vi "诊断标定3 - 副本.vi"(8 "CAN端口":u16(ring), 9 "设备索引号":u16(ring), 10 "CAN卡类型":u32(ring)=21) -> ()   [LabVIEW 2013] (continued)
                n961 = property on="项目信息" class="Tbl (严格)"("Disabled"=w1279) -> ()  [unwired: 2 in, 2 out]
                n962 = global read "功能码全局.vi" "主板项目信息5"() -> (w1287:bool[])
                n963 = global read "功能码全局.vi" "主板项目信息6"() -> (w1285:bool[])
                n964 = Index Array(array=w1287, index=4 ("索引")) -> (element=w1283:bool)
                n965 = Index Array(array=w1285, index=5 ("索引")) -> (element=w1284:bool)
                n966 = Not(x=w1293) -> (.not. x?=w1292:bool)
              }
              frame "温度起始值" {
                w1329 = 2
                w1331 = FALSE
                n967 = property on="电池实际容量(A)" class="DigNum (严格)"("Disabled"=w1329) -> ()  [unwired: 2 in, 2 out]
                n968 = property on="使用者" class="DigNum (严格)"("Disabled"=w1329) -> ()  [unwired: 2 in, 2 out]
                n969 = property on="SOH(%)" class="DigNum (严格)"("Disabled"=w1329) -> ()  [unwired: 2 in, 2 out]
                n970 = property on="电池额定容量(A)" class="DigNum (严格)"("Disabled"=w1329) -> ()  [unwired: 2 in, 2 out]
                n971 = property on="SOC(%)" class="DigNum (严格)"("Disabled"=w1329) -> ()  [unwired: 2 in, 2 out]
                n972 = local read "从板个数"() -> (w1327:dbl)
                n973 = property on="系统时钟" class="Str"("Disabled"=w1329) -> ()  [unwired: 2 in, 2 out]
                n974 = property on="配置文件版本" class="Str"("Disabled"=w1329) -> ()  [unwired: 2 in, 2 out]
                n975 = property on="车架(牌)号" class="Str"("Disabled"=w1329) -> ()  [unwired: 2 in, 2 out]
                n976 = property on="产品编号" class="Str"("Disabled"=w1329) -> ()  [unwired: 2 in, 2 out]
                n977 = control-ref of="项目信息"() -> (w1328:refnum<vi>)
                n978 = stacked-sequence {
                  tunnel: w1328 -> [w1340 w1343 w1356]
                  tunnel: w1327 -> [w1333 w1342 w1355]
                  frame #0 {
                    n979 = Multiply(x=w1333, y=3.0) -> (x*y=w1335:dbl)
                    n980 = Compound Arithmetic op=ADD(23.0 ("值"), w1335) -> (w1337:dbl)
                    n981 = Bundle(w1337, 0) -> (w1339:cluster{dbl, i32})  [unwired: 1 out]
                    n982 = property class="Tbl (严格)"(reference=w1340, "Index Values"=w1339) -> ()  [unwired: 1 in, 2 out]
                  }
                  frame #1 {
                    n983 = for {
                      N: 10 -> [_]
                      tunnel: w1343 -> [w1353]
                      tunnel: w1342 -> [w1348]
                      i -> [w1347]
                      n984 = Multiply(x=4.0, y=w1348) -> (x*y=w1345:dbl)
                      n985 = Compound Arithmetic op=ADD(24.0 ("值"), w1345, w1347) -> (w1350:dbl)
                      n986 = Bundle(w1350, 0) -> (w1352:cluster{dbl, i32})  [unwired: 1 out]
                      n987 = property class="Tbl (严格)"(reference=w1353, "Active Cell"=w1352, "Cell BG Color"=u32 16448250) -> ()  [unwired: 1 in, 2 out]
                    }
                  }
                  frame #2 {
                    n988 = Increment(x=w1355) -> (x+1=w1354:dbl)
                    n989 = for {
                      N: w1354 -> [_]
                      tunnel: w1356 -> [w1366]
                      tunnel: w1355 -> [w1361]
                      i -> [w1360]
                      n990 = Multiply(x=3.0, y=w1361) -> (x*y=w1358:dbl)
                      n991 = Compound Arithmetic op=ADD(23.0 ("值"), w1358, w1360) -> (w1363:dbl)
                      n992 = Bundle(w1363, 0) -> (w1365:cluster{dbl, i32})  [unwired: 1 out]
                      n993 = property class="Tbl (严格)"(reference=w1366, "Active Cell"=w1365, "Cell BG Color"=u32 6618880) -> ()  [unwired: 1 in, 2 out]
                    }
                  }
                }
                n994 = Select(t=0, s=w1318, f=1) -> (s? t:f=w1317:i32)
                n995 = property on="从板个数" class="DigNum (严格)"("NumText.BGColor"=u32 13816530) -> ()  [unwired: 2 in, 2 out]
                n996 = property on="项目信息" class="Tbl (严格)"("Disabled"=w1317) -> ()  [unwired: 2 in, 2 out]
                n997 = global read "功能码全局.vi" "主板项目信息5"() -> (w1325:bool[])
                n998 = global read "功能码全局.vi" "主板项目信息6"() -> (w1323:bool[])
                n999 = Index Array(array=w1325, index=5 ("索引")) -> (element=w1322:bool)
                n1000 = Index Array(array=w1323, index=6 ("索引")) -> (element=w1321:bool)
                n1001 = Not(x=w1331) -> (.not. x?=w1330:bool)
              }
              frame "保险位置" {
                w1379 = 2
                w1381 = FALSE
                n1002 = property on="电池实际容量(A)" class="DigNum (严格)"("Disabled"=w1379) -> ()  [unwired: 2 in, 2 out]
                n1003 = property on="使用者" class="DigNum (严格)"("Disabled"=w1379) -> ()  [unwired: 2 in, 2 out]
                n1004 = property on="SOH(%)" class="DigNum (严格)"("Disabled"=w1379) -> ()  [unwired: 2 in, 2 out]
                n1005 = property on="电池额定容量(A)" class="DigNum (严格)"("Disabled"=w1379) -> ()  [unwired: 2 in, 2 out]
                n1006 = property on="SOC(%)" class="DigNum (严格)"("Disabled"=w1379) -> ()  [unwired: 2 in, 2 out]
                n1007 = local read "从板个数"() -> (w1377:dbl)
                n1008 = property on="系统时钟" class="Str"("Disabled"=w1379) -> ()  [unwired: 2 in, 2 out]
                n1009 = property on="配置文件版本" class="Str"("Disabled"=w1379) -> ()  [unwired: 2 in, 2 out]
                n1010 = property on="车架(牌)号" class="Str"("Disabled"=w1379) -> ()  [unwired: 2 in, 2 out]
                n1011 = property on="产品编号" class="Str"("Disabled"=w1379) -> ()  [unwired: 2 in, 2 out]
                n1012 = control-ref of="项目信息"() -> (w1378:refnum<vi>)
                n1013 = stacked-sequence {
                  tunnel: w1378 -> [w1390 w1393]
                  tunnel: w1377 -> [w1383 w1392]
                  frame #0 {
                    n1014 = Multiply(x=w1383, y=4.0) -> (x*y=w1385:dbl)
                    n1015 = Compound Arithmetic op=ADD(24.0 ("值"), w1385) -> (w1387:dbl)
                    n1016 = Bundle(w1387, 0) -> (w1389:cluster{dbl, i32})  [unwired: 1 out]
                    n1017 = property class="Tbl (严格)"(reference=w1390, "Index Values"=w1389) -> ()  [unwired: 1 in, 2 out]
                  }
                  frame #1 {
                    n1018 = for {
                      N: 20 -> [_]
                      tunnel: w1393 -> [w1403]
                      tunnel: w1392 -> [w1398]
                      i -> [w1397]
                      n1019 = Multiply(x=4.0, y=w1398) -> (x*y=w1395:dbl)
                      n1020 = Compound Arithmetic op=ADD(24.0 ("值"), w1395, w1397) -> (w1400:dbl)
                      n1021 = Bundle(w1400, 0) -> (w1402:cluster{dbl, i32})  [unwired: 1 out]
                      n1022 = property class="Tbl (严格)"(reference=w1403, "Active Cell"=w1402, "Cell BG Color"=u32 6618880) -> ()  [unwired: 1 in, 2 out]
                    }
                  }
                }
                n1023 = property on="从板个数" class="DigNum (严格)"("NumText.BGColor"=u32 13816530) -> ()  [unwired: 2 in, 2 out]
                n1024 = Select(t=0, s=w1370, f=1) -> (s? t:f=w1368:i32)
                n1025 = global read "功能码全局.vi" "主板项目信息4"() -> (w1375:bool[])
                n1026 = property on="项目信息" class="Tbl (严格)"("Disabled"=w1368) -> ()  [unwired: 2 in, 2 out]
                n1027 = Index Array(array=w1375, index #1=5 ("索引"), index #2=6 ("索引")) -> (element #1=w1373:bool, element #2=w1372:bool)
                n1028 = Not(x=w1381) -> (.not. x?=w1380:bool)
              }
              frame "SOC" {
                w1414 = 2
                w1416 = FALSE
                n1029 = property on="电池实际容量(A)" class="DigNum (严格)"("Disabled"=w1414) -> ()  [unwired: 2 in, 2 out]
                n1030 = property on="使用者" class="DigNum (严格)"("Disabled"=w1414) -> ()  [unwired: 2 in, 2 out]
                n1031 = property on="SOH(%)" class="DigNum (严格)"("Disabled"=w1414) -> ()  [unwired: 2 in, 2 out]
                n1032 = property on="电池额定容量(A)" class="DigNum (严格)"("Disabled"=w1414) -> ()  [unwired: 2 in, 2 out]
                n1033 = property on="从板个数" class="DigNum (严格)"("NumText.BGColor"=u32 13816530) -> ()  [unwired: 2 in, 2 out]
                n1034 = property on="系统时钟" class="Str"("Disabled"=w1414) -> ()  [unwired: 2 in, 2 out]
                n1035 = property on="配置文件版本" class="Str"("Disabled"=w1414) -> ()  [unwired: 2 in, 2 out]
                n1036 = property on="车架(牌)号" class="Str"("Disabled"=w1414) -> ()  [unwired: 2 in, 2 out]
                n1037 = property on="项目信息" class="Tbl (严格)"("Disabled"=w1414) -> ()  [unwired: 2 in, 2 out]
                n1038 = property on="产品编号" class="Str"("Disabled"=w1414) -> ()  [unwired: 2 in, 2 out]
                n1039 = Select(t=0, s=w1406, f=0) -> (s? t:f=w1405:i32)
                n1040 = property on="SOC(%)" class="DigNum (严格)"("Disabled"=w1405) -> ()  [unwired: 2 in, 2 out]
                n1041 = property on="项目信息2" class="Clust (严格)"("DisabledEnum"=w1405) -> ()  [unwired: 2 in, 2 out]
                n1042 = global read "功能码全局.vi" "主板项目信息7"() -> (w1412:bool[])
                n1043 = Index Array(array=w1412, index #1=2 ("索引"), index #2=5 ("索引")) -> (element #1=w1410:bool, element #2=w1409:bool)
                n1044 = Not(x=w1416) -> (.not. x?=w1415:bool)
              }
              frame "电池额定实际容量" {
                w1428 = 2
                w1430 = FALSE
                n1045 = property on="使用者" class="DigNum (严格)"("Disabled"=w1428) -> ()  [unwired: 2 in, 2 out]
                n1046 = property on="SOH(%)" class="DigNum (严格)"("Disabled"=w1428) -> ()  [unwired: 2 in, 2 out]
                n1047 = property on="SOC(%)" class="DigNum (严格)"("Disabled"=w1428) -> ()  [unwired: 2 in, 2 out]
                n1048 = property on="从板个数" class="DigNum (严格)"("NumText.BGColor"=u32 13816530) -> ()  [unwired: 2 in, 2 out]
                n1049 = property on="系统时钟" class="Str"("Disabled"=w1428) -> ()  [unwired: 2 in, 2 out]
                n1050 = property on="配置文件版本" class="Str"("Disabled"=w1428) -> ()  [unwired: 2 in, 2 out]
                n1051 = property on="车架(牌)号" class="Str"("Disabled"=w1428) -> ()  [unwired: 2 in, 2 out]
                n1052 = property on="项目信息" class="Tbl (严格)"("Disabled"=w1428) -> ()  [unwired: 2 in, 2 out]
                n1053 = property on="产品编号" class="Str"("Disabled"=w1428) -> ()  [unwired: 2 in, 2 out]
                n1054 = Select(t=0, s=w1420, f=1) -> (s? t:f=w1419:i32)
                n1055 = property on="电池实际容量(A)" class="DigNum (严格)"("Disabled"=w1419) -> ()  [unwired: 2 in, 2 out]
                n1056 = property on="电池额定容量(A)" class="DigNum (严格)"("Disabled"=w1419) -> ()  [unwired: 2 in, 2 out]
                n1057 = property on="项目信息2" class="Clust (严格)"("DisabledEnum"=w1419) -> ()  [unwired: 2 in, 2 out]
                n1058 = global read "功能码全局.vi" "主板项目信息7"() -> (w1426:bool[])
                n1059 = Index Array(array=w1426, index #1=3 ("索引"), index #2=6 ("索引")) -> (element #1=w1424:bool, element #2=w1423:bool)
                n1060 = Not(x=w1430) -> (.not. x?=w1429:bool)
              }
              frame "配置文件版本" {
                w1443 = 2
                w1445 = FALSE
                n1061 = property on="使用者" class="DigNum (严格)"("Disabled"=w1443) -> ()  [unwired: 2 in, 2 out]
                n1062 = property on="SOH(%)" class="DigNum (严格)"("Disabled"=w1443) -> ()  [unwired: 2 in, 2 out]
                n1063 = property on="SOC(%)" class="DigNum (严格)"("Disabled"=w1443) -> ()  [unwired: 2 in, 2 out]
                n1064 = property on="电池实际容量(A)" class="DigNum (严格)"("Disabled"=w1443) -> ()  [unwired: 2 in, 2 out]
                n1065 = property on="从板个数" class="DigNum (严格)"("NumText.BGColor"=u32 13816530) -> ()  [unwired: 2 in, 2 out]
                n1066 = property on="电池额定容量(A)" class="DigNum (严格)"("Disabled"=w1443) -> ()  [unwired: 2 in, 2 out]
                n1067 = property on="系统时钟" class="Str"("Disabled"=w1443) -> ()  [unwired: 2 in, 2 out]
                n1068 = property on="车架(牌)号" class="Str"("Disabled"=w1443) -> ()  [unwired: 2 in, 2 out]
                n1069 = property on="项目信息" class="Tbl (严格)"("Disabled"=w1443) -> ()  [unwired: 2 in, 2 out]
                n1070 = property on="产品编号" class="Str"("Disabled"=w1443) -> ()  [unwired: 2 in, 2 out]
                n1071 = Select(t=0, s=w1434, f=1) -> (s? t:f=w1433:i32)
                n1072 = property on="项目信息2" class="Clust (严格)"("DisabledEnum"=w1433) -> ()  [unwired: 2 in, 2 out]
                n1073 = property on="配置文件版本" class="Str"("Disabled"=w1433) -> ()  [unwired: 2 in, 2 out]
                n1074 = global read "功能码全局.vi" "主板项目信息5"() -> (w1441:bool[])
                n1075 = global read "功能码全局.vi" "主板项目信息6"() -> (w1440:bool[])
                n1076 = Index Array(array=w1441, index=6 ("索引")) -> (element=w1438:bool)
                n1077 = Index Array(array=w1440, index=7 ("索引")) -> (element=w1437:bool)
                n1078 = Not(x=w1445) -> (.not. x?=w1444:bool)
              }
              frame "参数修改记录" {
                w1458 = 2
                w1460 = FALSE
                n1079 = property on="SOH(%)" class="DigNum (严格)"("Disabled"=w1458) -> ()  [unwired: 2 in, 2 out]
                n1080 = property on="SOC(%)" class="DigNum (严格)"("Disabled"=w1458) -> ()  [unwired: 2 in, 2 out]
                n1081 = property on="电池实际容量(A)" class="DigNum (严格)"("Disabled"=w1458) -> ()  [unwired: 2 in, 2 out]
                n1082 = property on="电池额定容量(A)" class="DigNum (严格)"("Disabled"=w1458) -> ()  [unwired: 2 in, 2 out]
                n1083 = property on="从板个数" class="DigNum (严格)"("NumText.BGColor"=u32 13816530) -> ()  [unwired: 2 in, 2 out]
                n1084 = property on="系统时钟" class="Str"("Disabled"=w1458) -> ()  [unwired: 2 in, 2 out]
                n1085 = property on="车架(牌)号" class="Str"("Disabled"=w1458) -> ()  [unwired: 2 in, 2 out]
                n1086 = property on="配置文件版本" class="Str"("Disabled"=w1458) -> ()  [unwired: 2 in, 2 out]
                n1087 = property on="项目信息" class="Tbl (严格)"("Disabled"=w1458) -> ()  [unwired: 2 in, 2 out]
                n1088 = property on="产品编号" class="Str"("Disabled"=w1458) -> ()  [unwired: 2 in, 2 out]
                n1089 = Select(t=0, s=w1449, f=1) -> (s? t:f=w1448:i32)
                n1090 = property on="使用者" class="DigNum (严格)"("Disabled"=w1448) -> ()  [unwired: 2 in, 2 out]
                n1091 = property on="项目信息2" class="Clust (严格)"("DisabledEnum"=w1448) -> ()  [unwired: 2 in, 2 out]
                n1092 = global read "功能码全局.vi" "主板项目信息7"() -> (w1455:bool[])
                n1093 = global read "功能码全局.vi" "主板项目信息5"() -> (w1456:bool[])
                n1094 = Index Array(array=w1455, index=0 ("索引")) -> (element=w1453:bool)
                n1095 = Index Array(array=w1456, index=7 ("索引")) -> (element=w1452:bool)
                n1096 = Not(x=w1460) -> (.not. x?=w1459:bool)
              }
              frame "车牌号" {
                w1473 = 2
                w1475 = FALSE
                n1097 = property on="SOH(%)" class="DigNum (严格)"("Disabled"=w1473) -> ()  [unwired: 2 in, 2 out]
                n1098 = property on="使用者" class="DigNum (严格)"("Disabled"=w1473) -> ()  [unwired: 2 in, 2 out]
                n1099 = property on="SOC(%)" class="DigNum (严格)"("Disabled"=w1473) -> ()  [unwired: 2 in, 2 out]
                n1100 = property on="电池实际容量(A)" class="DigNum (严格)"("Disabled"=w1473) -> ()  [unwired: 2 in, 2 out]
                n1101 = property on="电池额定容量(A)" class="DigNum (严格)"("Disabled"=w1473) -> ()  [unwired: 2 in, 2 out]
                n1102 = property on="从板个数" class="DigNum (严格)"("NumText.BGColor"=u32 13816530) -> ()  [unwired: 2 in, 2 out]
                n1103 = property on="系统时钟" class="Str"("Disabled"=w1473) -> ()  [unwired: 2 in, 2 out]
                n1104 = property on="配置文件版本" class="Str"("Disabled"=w1473) -> ()  [unwired: 2 in, 2 out]
                n1105 = property on="项目信息" class="Tbl (严格)"("Disabled"=w1473) -> ()  [unwired: 2 in, 2 out]
                n1106 = property on="产品编号" class="Str"("Disabled"=w1473) -> ()  [unwired: 2 in, 2 out]
                n1107 = Select(t=0, s=w1464, f=1) -> (s? t:f=w1463:i32)
                n1108 = property on="车架(牌)号" class="Str"("Disabled"=w1463) -> ()  [unwired: 2 in, 2 out]
                n1109 = property on="项目信息2" class="Clust (严格)"("DisabledEnum"=w1463) -> ()  [unwired: 2 in, 2 out]
                n1110 = global read "功能码全局.vi" "主板项目信息7"() -> (w1470:bool[])
                n1111 = global read "功能码全局.vi" "主板项目信息6"() -> (w1471:bool[])
                n1112 = Index Array(array=w1470, index=1 ("索引")) -> (element=w1468:bool)
                n1113 = Index Array(array=w1471, index=0 ("索引")) -> (element=w1467:bool)
                n1114 = Not(x=w1475) -> (.not. x?=w1474:bool)
              }
              frame "SOH" {
                w1487 = 2
                w1489 = FALSE
                n1115 = property on="使用者" class="DigNum (严格)"("Disabled"=w1487) -> ()  [unwired: 2 in, 2 out]
                n1116 = property on="SOC(%)" class="DigNum (严格)"("Disabled"=w1487) -> ()  [unwired: 2 in, 2 out]
                n1117 = property on="电池实际容量(A)" class="DigNum (严格)"("Disabled"=w1487) -> ()  [unwired: 2 in, 2 out]
                n1118 = property on="电池额定容量(A)" class="DigNum (严格)"("Disabled"=w1487) -> ()  [unwired: 2 in, 2 out]
                n1119 = property on="从板个数" class="DigNum (严格)"("NumText.BGColor"=u32 13816530) -> ()  [unwired: 2 in, 2 out]
                n1120 = property on="系统时钟" class="Str"("Disabled"=w1487) -> ()  [unwired: 2 in, 2 out]
                n1121 = property on="配置文件版本" class="Str"("Disabled"=w1487) -> ()  [unwired: 2 in, 2 out]
                n1122 = property on="项目信息" class="Tbl (严格)"("Disabled"=w1487) -> ()  [unwired: 2 in, 2 out]
                n1123 = property on="产品编号" class="Str"("Disabled"=w1487) -> ()  [unwired: 2 in, 2 out]
                n1124 = property on="车架(牌)号" class="Str"("Disabled"=w1487) -> ()  [unwired: 2 in, 2 out]
                n1125 = Select(t=0, s=w1479, f=1) -> (s? t:f=w1478:i32)
                n1126 = property on="项目信息2" class="Clust (严格)"("DisabledEnum"=w1478) -> ()  [unwired: 2 in, 2 out]
                n1127 = property on="SOH(%)" class="DigNum (严格)"("Disabled"=w1478) -> ()  [unwired: 2 in, 2 out]
                n1128 = global read "功能码全局.vi" "主板项目信息7"() -> (w1486:bool[])
                n1129 = Index Array(array=w1486, index #1=4 ("索引"), index #2=7 ("索引")) -> (element #1=w1483:bool, element #2=w1482:bool)
                n1130 = Not(x=w1489) -> (.not. x?=w1488:bool)
              }
              frame "SOC过低(2)", "SOC过高(2)", "SOH过低(2)", "充电电流过高(2)", "单体电压过低(2)", "单体电压过高(2)", "单组电压不均衡(2)", "单组温度不均衡(2)", "二级故障阀值", "放电电流过高(2)", "极柱温度过高(2)", "内阻过大(2)", "温度过低(2)", "温度过高(2)", "整组电压不均衡(2)", "整组温度不均衡(2)", "总电压过低(2)", "总电压过高(2)" {
                w1501 = FALSE
                n1131 = property on="从板个数" class="DigNum (严格)"("NumText.BGColor"=u32 13816530) -> ()  [unwired: 2 in, 2 out]
                n1132 = Select(t=0, s=w1493, f=1) -> (s? t:f=w1492:i32)
                n1133 = property on="一级故障 2" class="Clust (严格)"("DisabledEnum"=w1492) -> ()  [unwired: 2 in, 2 out]
                n1134 = global read "功能码全局.vi" "主板故障阀值9"() -> (w1499:bool[])
                n1135 = Index Array(array=w1499, index #1=3 ("索引"), index #2=6 ("索引")) -> (element #1=w1497:bool, element #2=w1496:bool)
                n1136 = Not(x=w1501) -> (.not. x?=w1502:bool)
              }
              frame "SOC过低(3)", "SOC过高(3)", "SOH过低(3)", "充电电流过高(3)", "单体电压过低(3)", "单体电压过高(3)", "单组电压不均衡(3)", "单组温度不均衡(3)", "放电电流过高(3)", "极柱温度过高(3)", "内阻过大(3)", "三级故障阀值", "温度过低(3)", "温度过高(3)", "整组电压不均衡(3)", "整组温度不均衡(3)", "总电压过低(3)", "总电压过高(3)" {
                w1515 = FALSE
                n1137 = property on="从板个数" class="DigNum (严格)"("NumText.BGColor"=u32 13816530) -> ()  [unwired: 2 in, 2 out]
                n1138 = Select(t=0, s=w1506, f=1) -> (s? t:f=w1505:i32)
                n1139 = property on="一级故障 3" class="Clust (严格)"("DisabledEnum"=w1505) -> ()  [unwired: 2 in, 2 out]
                n1140 = global read "功能码全局.vi" "主板故障阀值9"() -> (w1512:bool[])
                n1141 = Index Array(array=w1512, index #1=4 ("索引"), index #2=7 ("索引")) -> (element #1=w1510:bool, element #2=w1509:bool)
                n1142 = Not(x=w1515) -> (.not. x?=w1514:bool)
              }
              frame "SOC过低", "SOC过高", "SOH过低", "充电电流过高", "单体电压过低", "单体电压过高", "单组电压不均衡", "单组温度不均衡", "放电电流过高", "极柱温度过高", "内阻过大", "温度过低", "温度过高", "一级故障阀值", "整组电压不均衡", "整组温度不均衡", "总电压过低", "总电压过高" {
                w1528 = FALSE
                n1143 = Select(t=0, s=w1519, f=1) -> (s? t:f=w1518:i32)
                n1144 = property on="从板个数" class="DigNum (严格)"("NumText.BGColor"=u32 13816530) -> ()  [unwired: 2 in, 2 out]
                n1145 = property on="一级故障" class="Clust (严格)"("DisabledEnum"=w1518) -> ()  [unwired: 2 in, 2 out]
                n1146 = global read "功能码全局.vi" "主板故障阀值9"() -> (w1525:bool[])
                n1147 = Index Array(array=w1525, index #1=2 ("索引"), index #2=5 ("索引")) -> (element #1=w1523:bool, element #2=w1522:bool)
                n1148 = Not(x=w1528) -> (.not. x?=w1527:bool)
              }
              frame "充电控制参数", "电流步长", "最大允许充电电流", "最大允许充电温度", "最大允许单体电压", "最大允许总电压", "最小允许充电电流", "最小允许充电温度", "最小允许单体电压" {
                w1531 = 2
                w1542 = FALSE
                n1149 = property on="从板个数" class="DigNum (严格)"("NumText.BGColor"=u32 13816530) -> ()  [unwired: 2 in, 2 out]
                n1150 = property on="风机开启温度" class="DigNum (严格)"("Disabled"=w1531) -> ()  [unwired: 2 in, 2 out]
                n1151 = property on="风机关闭温度" class="DigNum (严格)"("Disabled"=w1531) -> ()  [unwired: 2 in, 2 out]
                n1152 = property on="加热开启温度" class="DigNum (严格)"("Disabled"=w1531) -> ()  [unwired: 2 in, 2 out]
                n1153 = property on="加热关闭温度" class="DigNum (严格)"("Disabled"=w1531) -> ()  [unwired: 2 in, 2 out]
                n1154 = property on="风机开启温差" class="DigNum (严格)"("Disabled"=w1531) -> ()  [unwired: 2 in, 2 out]
                n1155 = property on="风机关闭温差" class="DigNum (严格)"("Disabled"=w1531) -> ()  [unwired: 2 in, 2 out]
                n1156 = property on="加热控制参数" class="Clust (严格)"("DisabledEnum"=w1531) -> ()  [unwired: 2 in, 2 out]
                n1157 = Select(t=0, s=w1533, f=1) -> (s? t:f=w1532:i32)
                n1158 = property on="最大允许总电压" class="DigNum (严格)"("Disabled"=w1532) -> ()  [unwired: 2 in, 2 out]
                n1159 = property on="最大允许充电温度" class="DigNum (严格)"("Disabled"=w1532) -> ()  [unwired: 2 in, 2 out]
                n1160 = property on="最小允许充电温度" class="DigNum (严格)"("Disabled"=w1532) -> ()  [unwired: 2 in, 2 out]
                n1161 = property on="电流步长" class="DigNum (严格)"("Disabled"=w1532) -> ()  [unwired: 2 in, 2 out]
                n1162 = property on="最大允许单体电压" class="DigNum (严格)"("Disabled"=w1532) -> ()  [unwired: 2 in, 2 out]
                n1163 = property on="最小允许单体电压" class="DigNum (严格)"("Disabled"=w1532) -> ()  [unwired: 2 in, 2 out]
                n1164 = property on="最大允许充电电流" class="DigNum (严格)"("Disabled"=w1532) -> ()  [unwired: 2 in, 2 out]
                n1165 = property on="最小允许充电电流" class="DigNum (严格)"("Disabled"=w1532) -> ()  [unwired: 2 in, 2 out]
                n1166 = global read "功能码全局.vi" "主板控制类信息10"() -> (w1539:bool[])
                n1167 = Index Array(array=w1539, index #1=5 ("索引"), index #2=7 ("索引")) -> (element #1=w1537:bool, element #2=w1536:bool)
                n1168 = Not(x=w1542) -> (.not. x?=w1541:bool)
              }
              frame "风机关闭温差", "风机关闭温度", "风机开启温差", "风机开启温度", "加热关闭温差", "加热关闭温度", "加热开启温度", "加热控制参数" {
                w1554 = 2
                w1556 = FALSE
                n1169 = Select(t=0, s=w1546, f=1) -> (s? t:f=w1545:i32)
                n1170 = property on="从板个数" class="DigNum (严格)"("NumText.BGColor"=u32 13816530) -> ()  [unwired: 2 in, 2 out]
                n1171 = property on="加热控制参数" class="Clust (严格)"("DisabledEnum"=w1545) -> ()  [unwired: 2 in, 2 out]
                n1172 = property on="风机开启温度" class="DigNum (严格)"("Disabled"=w1545) -> ()  [unwired: 2 in, 2 out]
                n1173 = property on="风机关闭温度" class="DigNum (严格)"("Disabled"=w1545) -> ()  [unwired: 2 in, 2 out]
                n1174 = property on="加热开启温度" class="DigNum (严格)"("Disabled"=w1545) -> ()  [unwired: 2 in, 2 out]
                n1175 = property on="加热关闭温度" class="DigNum (严格)"("Disabled"=w1545) -> ()  [unwired: 2 in, 2 out]
                n1176 = property on="风机开启温差" class="DigNum (严格)"("Disabled"=w1545) -> ()  [unwired: 2 in, 2 out]
                n1177 = property on="风机关闭温差" class="DigNum (严格)"("Disabled"=w1545) -> ()  [unwired: 2 in, 2 out]
                n1178 = property on="最大允许总电压" class="DigNum (严格)"("Disabled"=w1554) -> ()  [unwired: 2 in, 2 out]
                n1179 = property on="最大允许充电温度" class="DigNum (严格)"("Disabled"=w1554) -> ()  [unwired: 2 in, 2 out]
                n1180 = property on="最小允许充电温度" class="DigNum (严格)"("Disabled"=w1554) -> ()  [unwired: 2 in, 2 out]
                n1181 = property on="电流步长" class="DigNum (严格)"("Disabled"=w1554) -> ()  [unwired: 2 in, 2 out]
                n1182 = property on="最大允许单体电压" class="DigNum (严格)"("Disabled"=w1554) -> ()  [unwired: 2 in, 2 out]
                n1183 = property on="最小允许单体电压" class="DigNum (严格)"("Disabled"=w1554) -> ()  [unwired: 2 in, 2 out]
                n1184 = property on="最大允许充电电流" class="DigNum (严格)"("Disabled"=w1554) -> ()  [unwired: 2 in, 2 out]
                n1185 = property on="最小允许充电电流" class="DigNum (严格)"("Disabled"=w1554) -> ()  [unwired: 2 in, 2 out]
                n1186 = global read "功能码全局.vi" "主板控制类信息10"() -> (w1552:bool[])
                n1187 = Index Array(array=w1552, index #1=4 ("索引"), index #2=6 ("索引")) -> (element #1=w1550:bool, element #2=w1549:bool)
                n1188 = Not(x=w1556) -> (.not. x?=w1555:bool)
              }
              frame "电池信息" {
                w1569 = FALSE
                n1189 = Select(t=0, s=w1560, f=1) -> (s? t:f=w1559:i32)
                n1190 = property on="电池串联" class="DigNum (严格)"("Disabled"=w1559) -> ()  [unwired: 2 in, 2 out]
                n1191 = property on="电池并联" class="DigNum (严格)"("Disabled"=w1559) -> ()  [unwired: 2 in, 2 out]
                n1192 = property on="电池包额定容量" class="DigNum (严格)"("Disabled"=w1559) -> ()  [unwired: 2 in, 2 out]
                n1193 = property on="电池包额定能量(kWh)" class="DigNum (严格)"("Disabled"=w1559) -> ()  [unwired: 2 in, 2 out]
                n1194 = property on="电池包额定总电压" class="DigNum (严格)"("Disabled"=w1559) -> ()  [unwired: 2 in, 2 out]
                n1195 = property on="实际容量" class="DigNum (严格)"("Disabled"=w1559) -> ()  [unwired: 2 in, 2 out]
                n1196 = property on="电池包组号" class="Str"("Disabled"=w1559) -> ()  [unwired: 2 in, 2 out]
                n1197 = property on="电池生产日期" class="Str"("Disabled"=w1559) -> ()  [unwired: 2 in, 2 out]
                n1198 = property on="电池厂家" class="Str"("Disabled"=w1559) -> ()  [unwired: 2 in, 2 out]
                n1199 = property on="电池类型" class="Str"("Disabled"=w1559) -> ()  [unwired: 2 in, 2 out]
                n1200 = property on="累计充电总安时" class="DigNum (严格)"("Disabled"=w1559) -> ()  [unwired: 2 in, 2 out]
                n1201 = property on="累计放电总安时" class="DigNum (严格)"("Disabled"=w1559) -> ()  [unwired: 2 in, 2 out]
                n1202 = property on="电池放空次数" class="DigNum (严格)"("Disabled"=w1559) -> ()  [unwired: 2 in, 2 out]
                n1203 = property on="电池充满次数" class="DigNum (严格)"("Disabled"=w1559) -> ()  [unwired: 2 in, 2 out]
                n1204 = property on="电池充电次数" class="DigNum (严格)"("Disabled"=w1559) -> ()  [unwired: 2 in, 2 out]
                n1205 = property on="电池信息" class="Clust (严格)"("DisabledEnum"=w1559) -> ()  [unwired: 2 in, 2 out]
                n1206 = global read "功能码全局.vi" "主板版本号11"() -> (w1566:bool[])
                n1207 = property on="从板个数" class="DigNum (严格)"("NumText.BGColor"=u32 13816530) -> ()  [unwired: 2 in, 2 out]
                n1208 = Index Array(array=w1566, index #1=0 ("索引"), index #2=1 ("索引")) -> (element #1=w1564:bool, element #2=w1563:bool)
                n1209 = Not(x=w1569) -> (.not. x?=w1568:bool)
              }
              frame "电池信息1" {
                w1581 = 2
                w1583 = FALSE
                n1210 = Select(t=0, s=w1573, f=1) -> (s? t:f=w1572:i32)
                n1211 = property on="电池信息" class="Clust (严格)"("DisabledEnum"=w1572) -> ()  [unwired: 2 in, 2 out]
                n1212 = property on="电池生产日期" class="Str"("Disabled"=w1572) -> ()  [unwired: 2 in, 2 out]
                n1213 = property on="电池厂家" class="Str"("Disabled"=w1572) -> ()  [unwired: 2 in, 2 out]
                n1214 = property on="电池类型" class="Str"("Disabled"=w1572) -> ()  [unwired: 2 in, 2 out]
                n1215 = property on="电池串联" class="DigNum (严格)"("Disabled"=w1572) -> ()  [unwired: 2 in, 2 out]
                n1216 = property on="电池并联" class="DigNum (严格)"("Disabled"=w1572) -> ()  [unwired: 2 in, 2 out]
                n1217 = property on="电池包额定容量" class="DigNum (严格)"("Disabled"=w1572) -> ()  [unwired: 2 in, 2 out]
                n1218 = property on="电池包额定能量(kWh)" class="DigNum (严格)"("Disabled"=w1572) -> ()  [unwired: 2 in, 2 out]
                n1219 = property on="电池包额定总电压" class="DigNum (严格)"("Disabled"=w1572) -> ()  [unwired: 2 in, 2 out]
                n1220 = property on="实际容量" class="DigNum (严格)"("Disabled"=w1572) -> ()  [unwired: 2 in, 2 out]
                n1221 = property on="累计充电总安时" class="DigNum (严格)"("Disabled"=w1581) -> ()  [unwired: 2 in, 2 out]
                n1222 = property on="累计放电总安时" class="DigNum (严格)"("Disabled"=w1581) -> ()  [unwired: 2 in, 2 out]
                n1223 = property on="电池放空次数" class="DigNum (严格)"("Disabled"=w1581) -> ()  [unwired: 2 in, 2 out]
                n1224 = property on="电池充满次数" class="DigNum (严格)"("Disabled"=w1581) -> ()  [unwired: 2 in, 2 out]
                n1225 = property on="电池充电次数" class="DigNum (严格)"("Disabled"=w1581) -> ()  [unwired: 2 in, 2 out]
                n1226 = property on="从板个数" class="DigNum (严格)"("NumText.BGColor"=u32 13816530) -> ()  [unwired: 2 in, 2 out]
                n1227 = property on="电池包组号" class="Str"("Disabled"=w1581) -> ()  [unwired: 2 in, 2 out]
                n1228 = global read "功能码全局.vi" "主板版本号11"() -> (w1579:bool[])
                n1229 = Index Array(array=w1579, index #1=0 ("索引"), index #2=1 ("索引")) -> (element #1=w1577:bool, element #2=w1576:bool)
                n1230 = Not(x=w1583) -> (.not. x?=w1582:bool)
              }
              frame "电池包组号" {
                w1595 = 2
                w1597 = FALSE
                n1231 = property on="电池生产日期" class="Str"("Disabled"=w1595) -> ()  [unwired: 2 in, 2 out]
                n1232 = property on="电池厂家" class="Str"("Disabled"=w1595) -> ()  [unwired: 2 in, 2 out]
                n1233 = property on="电池类型" class="Str"("Disabled"=w1595) -> ()  [unwired: 2 in, 2 out]
                n1234 = property on="电池串联" class="DigNum (严格)"("Disabled"=w1595) -> ()  [unwired: 2 in, 2 out]
                n1235 = property on="电池并联" class="DigNum (严格)"("Disabled"=w1595) -> ()  [unwired: 2 in, 2 out]
                n1236 = property on="电池包额定容量" class="DigNum (严格)"("Disabled"=w1595) -> ()  [unwired: 2 in, 2 out]
                n1237 = property on="电池包额定能量(kWh)" class="DigNum (严格)"("Disabled"=w1595) -> ()  [unwired: 2 in, 2 out]
                n1238 = property on="电池包额定总电压" class="DigNum (严格)"("Disabled"=w1595) -> ()  [unwired: 2 in, 2 out]
                n1239 = property on="实际容量" class="DigNum (严格)"("Disabled"=w1595) -> ()  [unwired: 2 in, 2 out]
                n1240 = property on="从板个数" class="DigNum (严格)"("NumText.BGColor"=u32 13816530) -> ()  [unwired: 2 in, 2 out]
                n1241 = property on="累计充电总安时" class="DigNum (严格)"("Disabled"=w1595) -> ()  [unwired: 2 in, 2 out]
                n1242 = property on="累计放电总安时" class="DigNum (严格)"("Disabled"=w1595) -> ()  [unwired: 2 in, 2 out]
                n1243 = property on="电池放空次数" class="DigNum (严格)"("Disabled"=w1595) -> ()  [unwired: 2 in, 2 out]
                n1244 = property on="电池充满次数" class="DigNum (严格)"("Disabled"=w1595) -> ()  [unwired: 2 in, 2 out]
                n1245 = property on="电池充电次数" class="DigNum (严格)"("Disabled"=w1595) -> ()  [unwired: 2 in, 2 out]
                n1246 = Select(t=0, s=w1587, f=1) -> (s? t:f=w1586:i32)
                n1247 = property on="电池包组号" class="Str"("Disabled"=w1586) -> ()  [unwired: 2 in, 2 out]
                n1248 = property on="电池信息" class="Clust (严格)"("DisabledEnum"=w1586) -> ()  [unwired: 2 in, 2 out]
                n1249 = global read "功能码全局.vi" "主板版本号11"() -> (w1593:bool[])
                n1250 = Index Array(array=w1593, index #1=0 ("索引"), index #2=1 ("索引")) -> (element #1=w1591:bool, element #2=w1590:bool)
                n1251 = Not(x=w1597) -> (.not. x?=w1596:bool)
              }
              frame "充放电安时" {
                w1609 = 2
                w1611 = FALSE
                n1252 = property on="电池生产日期" class="Str"("Disabled"=w1609) -> ()  [unwired: 2 in, 2 out]
                n1253 = property on="电池厂家" class="Str"("Disabled"=w1609) -> ()  [unwired: 2 in, 2 out]
                n1254 = property on="电池类型" class="Str"("Disabled"=w1609) -> ()  [unwired: 2 in, 2 out]
                n1255 = property on="电池串联" class="DigNum (严格)"("Disabled"=w1609) -> ()  [unwired: 2 in, 2 out]
                n1256 = property on="电池并联" class="DigNum (严格)"("Disabled"=w1609) -> ()  [unwired: 2 in, 2 out]
                n1257 = property on="电池包额定容量" class="DigNum (严格)"("Disabled"=w1609) -> ()  [unwired: 2 in, 2 out]
                n1258 = property on="电池包额定能量(kWh)" class="DigNum (严格)"("Disabled"=w1609) -> ()  [unwired: 2 in, 2 out]
                n1259 = property on="电池包额定总电压" class="DigNum (严格)"("Disabled"=w1609) -> ()  [unwired: 2 in, 2 out]
                n1260 = property on="实际容量" class="DigNum (严格)"("Disabled"=w1609) -> ()  [unwired: 2 in, 2 out]
                n1261 = property on="从板个数" class="DigNum (严格)"("NumText.BGColor"=u32 13816530) -> ()  [unwired: 2 in, 2 out]
                n1262 = Select(t=0, s=w1601, f=1) -> (s? t:f=w1600:i32)
                n1263 = property on="电池放空次数" class="DigNum (严格)"("Disabled"=w1609) -> ()  [unwired: 2 in, 2 out]
                n1264 = property on="电池充满次数" class="DigNum (严格)"("Disabled"=w1609) -> ()  [unwired: 2 in, 2 out]
                n1265 = property on="电池充电次数" class="DigNum (严格)"("Disabled"=w1609) -> ()  [unwired: 2 in, 2 out]
                n1266 = property on="电池包组号" class="Str"("Disabled"=w1609) -> ()  [unwired: 2 in, 2 out]
                n1267 = property on="累计充电总安时" class="DigNum (严格)"("Disabled"=w1600) -> ()  [unwired: 2 in, 2 out]
                n1268 = property on="累计放电总安时" class="DigNum (严格)"("Disabled"=w1600) -> ()  [unwired: 2 in, 2 out]
                n1269 = property on="电池信息" class="Clust (严格)"("DisabledEnum"=w1600) -> ()  [unwired: 2 in, 2 out]
                n1270 = global read "功能码全局.vi" "主板版本号11"() -> (w1607:bool[])
                n1271 = Index Array(array=w1607, index #1=0 ("索引"), index #2=1 ("索引")) -> (element #1=w1605:bool, element #2=w1604:bool)
                n1272 = Not(x=w1611) -> (.not. x?=w1610:bool)
              }
              frame "电池充放电次数" {
                w1623 = 2
                w1625 = FALSE
                n1273 = property on="从板个数" class="DigNum (严格)"("NumText.BGColor"=u32 13816530) -> ()  [unwired: 2 in, 2 out]
                n1274 = property on="电池生产日期" class="Str"("Disabled"=w1623) -> ()  [unwired: 2 in, 2 out]
                n1275 = property on="电池厂家" class="Str"("Disabled"=w1623) -> ()  [unwired: 2 in, 2 out]
                n1276 = property on="电池类型" class="Str"("Disabled"=w1623) -> ()  [unwired: 2 in, 2 out]
                n1277 = property on="电池串联" class="DigNum (严格)"("Disabled"=w1623) -> ()  [unwired: 2 in, 2 out]
                n1278 = property on="电池并联" class="DigNum (严格)"("Disabled"=w1623) -> ()  [unwired: 2 in, 2 out]
                n1279 = property on="电池包额定容量" class="DigNum (严格)"("Disabled"=w1623) -> ()  [unwired: 2 in, 2 out]
                n1280 = property on="电池包额定能量(kWh)" class="DigNum (严格)"("Disabled"=w1623) -> ()  [unwired: 2 in, 2 out]
                n1281 = property on="电池包额定总电压" class="DigNum (严格)"("Disabled"=w1623) -> ()  [unwired: 2 in, 2 out]
                n1282 = property on="实际容量" class="DigNum (严格)"("Disabled"=w1623) -> ()  [unwired: 2 in, 2 out]
                n1283 = Select(t=0, s=w1615, f=1) -> (s? t:f=w1614:i32)
                n1284 = property on="电池放空次数" class="DigNum (严格)"("Disabled"=w1614) -> ()  [unwired: 2 in, 2 out]
                n1285 = property on="电池充满次数" class="DigNum (严格)"("Disabled"=w1614) -> ()  [unwired: 2 in, 2 out]
                n1286 = property on="电池充电次数" class="DigNum (严格)"("Disabled"=w1614) -> ()  [unwired: 2 in, 2 out]
                n1287 = property on="累计充电总安时" class="DigNum (严格)"("Disabled"=w1623) -> ()  [unwired: 2 in, 2 out]
                n1288 = property on="累计放电总安时" class="DigNum (严格)"("Disabled"=w1623) -> ()  [unwired: 2 in, 2 out]
                n1289 = property on="电池信息" class="Clust (严格)"("DisabledEnum"=w1614) -> ()  [unwired: 2 in, 2 out]
                n1290 = property on="电池包组号" class="Str"("Disabled"=w1623) -> ()  [unwired: 2 in, 2 out]
                n1291 = global read "功能码全局.vi" "主板版本号11"() -> (w1621:bool[])
                n1292 = Index Array(array=w1621, index #1=0 ("索引"), index #2=1 ("索引")) -> (element #1=w1619:bool, element #2=w1618:bool)
                n1293 = Not(x=w1625) -> (.not. x?=w1624:bool)
              }
              frame "假", Default {
                w1630 = FALSE
                n1294 = Not(x=w1630) -> (.not. x?=w1629:bool)
              }
            }
            n1295 = property on="单个读取" class="Bool (严格)"("Visible"=w1113) -> ()  [unwired: 2 in, 2 out]
            n1296 = property on="单个写入" class="Bool (严格)"("Visible"=w1112) -> ()  [unwired: 2 in, 2 out]
            n1297 = local write "1"(w1120) -> ()
            n1298 = local write "1 2"(w1119) -> ()
            n1299 = local write "1 3"(w1118) -> ()
            n1300 = local write "1 4"(w1117) -> ()
            n1301 = local write "1 5"(w1116) -> ()
            n1302 = local write "1 11"(w1115) -> ()
            n1303 = local write "主板2"(w1121) -> ()
          }
          event "从板选项": Mouse Down {
            n1304 = event-data() -> ("CtlRef"=w1645:refnum<vi>)  [unwired: 8 out]
            n1305 = property class="Tree (严格)"(reference=w1645) -> ("Value"=w1644:string)  [unwired: 1 in, 2 out]
            n1306 = global read "功能码全局.vi" "主板监控2"() -> (w1635:bool[])
            n1307 = Index Array(array=w1635, index=6 ("索引")) -> (element=w1633:bool)
            n1308 = case shown="\"温度个数\"" w1644 {
              tunnel: [T21."从板信息" ("等级 2") T21."从板信息" ("等级 2") T21."从板信息" ("等级 2") T21."从板信息" ("等级 2") T21."从板信息" ("等级 2") T21."从板信息" ("等级 2") T21."从板信息" ("等级 2") T21."一级故障阀值" ("等级 2") T21."二级故障阀值" ("等级 2") T21."三级故障阀值" ("等级 2") T21."快换参数" ("等级 2") T21."快换参数" ("等级 2") T21."快换参数" ("等级 2") T21."快换参数" ("等级 2") T21."快换参数" ("等级 2") T21."快换参数" ("等级 2") T21."快换参数" ("等级 2") T21."快换参数" ("等级 2") T14."均衡参数" ("等级 2") T14."均衡参数" ("等级 2") T14."均衡参数" ("等级 2") T21."从板信息" ("等级 2")] -> w1643
              tunnel: [w1656 w1666 w1680 w1695 w1730 w1767 w1804 w1828 w1841 w1854 w1867 w1893 w1907 w1923 w1940 w1957 w1975 w1994 w2011 w2024 w2038 w2053] -> w1642
              tunnel: [w1648 w1658 w1668 w1682 w1717 w1754 w1791 w1839 w1841 w1854 w1867 w1893 w1907 w1923 w1940 w1957 w1975 w1994 w2011 w2024 w2038 w2052] -> w1641
              tunnel: [w1648 w1658 w1668 w1682 w1717 w1754 w1791 w1828 w1852 w1854 w1867 w1893 w1907 w1923 w1940 w1957 w1975 w1994 w2011 w2024 w2038 w2052] -> w1640
              tunnel: [w1648 w1658 w1668 w1682 w1717 w1754 w1791 w1828 w1841 w1865 w1867 w1893 w1907 w1923 w1940 w1957 w1975 w1994 w2011 w2024 w2038 w2052] -> w1639
              tunnel: [w1648 w1658 w1668 w1682 w1717 w1754 w1791 w1828 w1841 w1854 w1891 w1905 w1921 w1938 w1955 w1973 w1992 w2009 w2011 w2024 w2038 w2052] -> w1638
              tunnel: [w1653 w1659 w1675 w1689 w1724 w1761 w1798 w1835 w1848 w1861 w1876 w1898 w1913 w1927 w1945 w1960 w1980 w1998 w2014 w2028 w2043 w2052] -> w1637
              tunnel: [w1650 w1659 w1674 w1688 w1723 w1760 w1797 w1834 w1847 w1860 w1868 w1897 w1912 w1926 w1946 w1961 w1979 w1997 w2013 w2027 w2042 w2052] -> w1636
              tunnel: w1633 -> [_ w1663 w1671 w1685 w1720 w1757 w1794 w1830 w1844 w1857 w1888 w1901 w1916 w1931 w1949 w1965 w1983 w2002 w2017 w2031 w2045 _]
              tunnel: [w1648 w1658 w1668 w1682 w1717 w1754 w1791 w1828 w1841 w1854 w1867 w1893 w1907 w1923 w1940 w1957 w1975 w1994 w2012 w2025 w2039 w2052] -> w1632
              frame "从板号" {
                w1655 = 2
                w1648 = FALSE ("1 6")
                n1309 = property on="项目信息 2" class="Tbl (严格)"("Disabled"=w1655) -> ()  [unwired: 2 in, 2 out]
                n1310 = property on="加热控制参数" class="Clust (严格)"("Disabled"=w1655) -> ()  [unwired: 2 in, 2 out]
                n1311 = property on="从板号" class="DigNum (严格)"("NumText.BGColor"=u32 6618880) -> ()  [unwired: 2 in, 2 out]
                n1312 = global read "功能码全局.vi" "16"() -> (w1652:bool[])
                n1313 = Index Array(array=w1652, index #1=4 ("索引"), index #2=6 ("索引")) -> (element #1=w1653:bool, element #2=w1650:bool)
                n1314 = Not(x=w1648) -> (.not. x?=w1656:bool)
              }
              frame "从板信息" {
                w1658 = FALSE ("1 6")
                n1315 = Select(t=0, s=w1663, f=1) -> (s? t:f=w1662:i32)
                n1316 = property on="从板号" class="DigNum (严格)"("NumText.BGColor"=u32 16777215) -> ()  [unwired: 2 in, 2 out]
                n1317 = property on="项目信息 2" class="Tbl (严格)"("Disabled"=w1662) -> ()  [unwired: 2 in, 2 out]
                n1318 = property on="加热控制参数" class="Clust (严格)"("Disabled"=w1662) -> ()  [unwired: 2 in, 2 out]
                n1319 = Not(x=w1658) -> (.not. x?=w1666:bool)
                n1320 = local read "从板项目信息"() -> (w1660:bool)
                n1321 = Not(x=w1660) -> (.not. x?=w1659:bool)
              }
              frame "风机关闭温差", "风机关闭温度", "风机开启温差", "风机开启温度", "加热关闭温差", "加热关闭温度", "加热开启温度", "加热控制参数" {
                w1668 = FALSE ("1 6")
                n1322 = property on="从板号" class="DigNum (严格)"("NumText.BGColor"=u32 16777215) -> ()  [unwired: 2 in, 2 out]
                n1323 = Select(t=0, s=w1671, f=1) -> (s? t:f=w1670:i32)
                n1324 = property on="项目信息 2" class="Tbl (严格)"("Disabled"=2) -> ()  [unwired: 2 in, 2 out]
                n1325 = property on="加热控制参数" class="Clust (严格)"("Disabled"=w1670) -> ()  [unwired: 2 in, 2 out]
                n1326 = global read "功能码全局.vi" "16"() -> (w1677:bool[])
                n1327 = Index Array(array=w1677, index #1=5 ("索引"), index #2=7 ("索引")) -> (element #1=w1675:bool, element #2=w1674:bool)
                n1328 = Not(x=w1668) -> (.not. x?=w1680:bool)
              }
              frame "电压个数" {
                w1682 = FALSE ("1 6")
                n1329 = property on="从板号" class="DigNum (严格)"("NumText.BGColor"=u32 16777215) -> ()  [unwired: 2 in, 2 out]
                n1330 = control-ref of="项目信息 2"() -> (w1693:refnum<vi>)
                n1331 = stacked-sequence {
                  tunnel: w1693 -> [w1700 w1702 w1711]
                  frame #0 {
                    n1332 = Bundle(0, 0) -> (w1699:cluster{i32, i32})  [unwired: 1 out]
                    n1333 = property class="Tbl (严格)"(reference=w1700, "Index Values"=w1699) -> ()  [unwired: 1 in, 2 out]
                  }
                  frame #1 {
                    n1334 = for {
                      N: 40 -> [_]
                      tunnel: w1702 -> [w1709]
                      i -> [w1704]
                      n1335 = Compound Arithmetic op=ADD(0 ("值"), w1704) -> (w1706:i32)
                      n1336 = Bundle(w1706, 0) -> (w1708:cluster{i32, i32})  [unwired: 1 out]
                      n1337 = property class="Tbl (严格)"(reference=w1709, "Active Cell"=w1708, "Cell BG Color"=u32 16448250) -> ()  [unwired: 1 in, 2 out]
                    }
                  }
                  frame #2 {
                    n1338 = for {
                      N: 1 -> [_]
                      tunnel: w1711 -> [w1716]
                      i -> [w1712]
                      n1339 = Bundle(w1712, 0) -> (w1715:cluster{i32, i32})  [unwired: 1 out]
                      n1340 = property class="Tbl (严格)"(reference=w1716, "Active Cell"=w1715, "Cell BG Color"=u32 6618880) -> ()  [unwired: 1 in, 2 out]
                    }
                  }
                }
                n1341 = Select(t=0, s=w1685, f=1) -> (s? t:f=w1684:i32)
                n1342 = property on="项目信息 2" class="Tbl (严格)"("Disabled"=w1684) -> ()  [unwired: 2 in, 2 out]
                n1343 = property on="加热控制参数" class="Clust (严格)"("Disabled"=2) -> ()  [unwired: 2 in, 2 out]
                n1344 = global read "功能码全局.vi" "15"() -> (w1691:bool[])
                n1345 = Index Array(array=w1691, index #1=0 ("索引"), index #2=4 ("索引")) -> (element #1=w1689:bool, element #2=w1688:bool)
                n1346 = Not(x=w1682) -> (.not. x?=w1695:bool)
              }
              frame "通道电压节数" {
                w1717 = FALSE ("1 6")
                n1347 = property on="从板号" class="DigNum (严格)"("NumText.BGColor"=u32 16777215) -> ()  [unwired: 2 in, 2 out]
                n1348 = control-ref of="项目信息 2"() -> (w1728:refnum<vi>)
                n1349 = stacked-sequence {
                  tunnel: w1728 -> [w1735 w1737 w1746]
                  frame #0 {
                    n1350 = Bundle(22, 0) -> (w1734:cluster{i32, i32})  [unwired: 1 out]
                    n1351 = property class="Tbl (严格)"(reference=w1735, "Index Values"=w1734) -> ()  [unwired: 1 in, 2 out]
                  }
                  frame #1 {
                    n1352 = for {
                      N: 40 -> [_]
                      tunnel: w1737 -> [w1744]
                      i -> [w1739]
                      n1353 = Compound Arithmetic op=ADD(0 ("值"), w1739) -> (w1741:i32)
                      n1354 = Bundle(w1741, 0) -> (w1743:cluster{i32, i32})  [unwired: 1 out]
                      n1355 = property class="Tbl (严格)"(reference=w1744, "Active Cell"=w1743, "Cell BG Color"=u32 16448250) -> ()  [unwired: 1 in, 2 out]
                    }
                  }
                  frame #2 {
                    n1356 = for {
                      N: 5 -> [_]
                      tunnel: w1746 -> [w1753]
                      i -> [w1749]
                      n1357 = Add(x=22, y=w1749) -> (x+y=w1748:i32)
                      n1358 = Bundle(w1748, 0) -> (w1752:cluster{i32, i32})  [unwired: 1 out]
                      n1359 = property class="Tbl (严格)"(reference=w1753, "Active Cell"=w1752, "Cell BG Color"=u32 6618880) -> ()  [unwired: 1 in, 2 out]
                    }
                  }
                }
                n1360 = Select(t=0, s=w1720, f=1) -> (s? t:f=w1719:i32)
                n1361 = property on="项目信息 2" class="Tbl (严格)"("Disabled"=w1719) -> ()  [unwired: 2 in, 2 out]
                n1362 = property on="加热控制参数" class="Clust (严格)"("Disabled"=2) -> ()  [unwired: 2 in, 2 out]
                n1363 = global read "功能码全局.vi" "15"() -> (w1726:bool[])
                n1364 = Index Array(array=w1726, index #1=1 ("索引"), index #2=5 ("索引")) -> (element #1=w1724:bool, element #2=w1723:bool)
                n1365 = Not(x=w1717) -> (.not. x?=w1730:bool)
              }
              frame "保险位置" {
                w1754 = FALSE ("1 6")
                n1366 = control-ref of="项目信息 2"() -> (w1765:refnum<vi>)
                n1367 = stacked-sequence {
                  tunnel: w1765 -> [w1772 w1774 w1783]
                  frame #0 {
                    n1368 = Bundle(0, 0) -> (w1771:cluster{i32, i32})  [unwired: 1 out]
                    n1369 = property class="Tbl (严格)"(reference=w1772, "Index Values"=w1771) -> ()  [unwired: 1 in, 2 out]
                  }
                  frame #1 {
                    n1370 = for {
                      N: 40 -> [_]
                      tunnel: w1774 -> [w1781]
                      i -> [w1777]
                      n1371 = Add(x=2, y=w1777) -> (x+y=w1776:i32)
                      n1372 = Bundle(w1776, 0) -> (w1780:cluster{i32, i32})  [unwired: 1 out]
                      n1373 = property class="Tbl (严格)"(reference=w1781, "Active Cell"=w1780, "Cell BG Color"=u32 16448250) -> ()  [unwired: 1 in, 2 out]
                    }
                  }
                  frame #2 {
                    n1374 = for {
                      N: 20 -> [_]
                      tunnel: w1783 -> [w1790]
                      i -> [w1786]
                      n1375 = Add(x=2, y=w1786) -> (x+y=w1785:i32)
                      n1376 = Bundle(w1785, 0) -> (w1789:cluster{i32, i32})  [unwired: 1 out]
                      n1377 = property class="Tbl (严格)"(reference=w1790, "Active Cell"=w1789, "Cell BG Color"=u32 6618880) -> ()  [unwired: 1 in, 2 out]
                    }
                  }
                }
                n1378 = property on="从板号" class="DigNum (严格)"("NumText.BGColor"=u32 16777215) -> ()  [unwired: 2 in, 2 out]
                n1379 = Select(t=0, s=w1757, f=1) -> (s? t:f=w1756:i32)
                n1380 = property on="项目信息 2" class="Tbl (严格)"("Disabled"=w1756) -> ()  [unwired: 2 in, 2 out]
                n1381 = property on="加热控制参数" class="Clust (严格)"("Disabled"=2) -> ()  [unwired: 2 in, 2 out]
                n1382 = global read "功能码全局.vi" "15"() -> (w1763:bool[])
                n1383 = Index Array(array=w1763, index #1=2 ("索引"), index #2=6 ("索引")) -> (element #1=w1761:bool, element #2=w1760:bool)
                n1384 = Not(x=w1754) -> (.not. x?=w1767:bool)
              }
              frame "温度个数" {
                w1791 = FALSE ("1 6")
                n1385 = control-ref of="项目信息 2"() -> (w1802:refnum<vi>)
                n1386 = stacked-sequence {
                  tunnel: w1802 -> [w1809 w1810 w1820]
                  frame #0 {
                    n1387 = Bundle(0, 0) -> (w1808:cluster{i32, i32})  [unwired: 1 out]
                    n1388 = property class="Tbl (严格)"(reference=w1809, "Index Values"=w1808) -> ()  [unwired: 1 in, 2 out]
                  }
                  frame #1 {
                    n1389 = for {
                      N: 40 -> [_]
                      tunnel: w1810 -> [w1818]
                      i -> [w1813]
                      n1390 = Compound Arithmetic op=ADD(0 ("值"), w1813) -> (w1815:i32)
                      n1391 = Bundle(w1815, 0) -> (w1817:cluster{i32, i32})  [unwired: 1 out]
                      n1392 = property class="Tbl (严格)"(reference=w1818, "Active Cell"=w1817, "Cell BG Color"=u32 16448250) -> ()  [unwired: 1 in, 2 out]
                    }
                  }
                  frame #2 {
                    n1393 = for {
                      N: 1 -> [_]
                      tunnel: w1820 -> [w1827]
                      i -> [w1823]
                      n1394 = Add(x=1, y=w1823) -> (x+y=w1822:i32)
                      n1395 = Bundle(w1822, 0) -> (w1826:cluster{i32, i32})  [unwired: 1 out]
                      n1396 = property class="Tbl (严格)"(reference=w1827, "Active Cell"=w1826, "Cell BG Color"=u32 6618880) -> ()  [unwired: 1 in, 2 out]
                    }
                  }
                }
                n1397 = Select(t=0, s=w1794, f=1) -> (s? t:f=w1793:i32)
                n1398 = property on="项目信息 2" class="Tbl (严格)"("Disabled"=w1793) -> ()  [unwired: 2 in, 2 out]
                n1399 = property on="加热控制参数" class="Clust (严格)"("Disabled"=2) -> ()  [unwired: 2 in, 2 out]
                n1400 = property on="从板号" class="DigNum (严格)"("NumText.BGColor"=u32 16777215) -> ()  [unwired: 2 in, 2 out]
                n1401 = global read "功能码全局.vi" "15"() -> (w1800:bool[])
                n1402 = Index Array(array=w1800, index #1=3 ("索引"), index #2=7 ("索引")) -> (element #1=w1798:bool, element #2=w1797:bool)
                n1403 = Not(x=w1791) -> (.not. x?=w1804:bool)
              }
              frame "SOC过低", "电压不均衡", "电压过低", "电压过高", "温度不均衡", "温度过低", "温度过高", "一级故障阀值" {
                w1828 = FALSE ("1 6")
                n1404 = property on="从板号" class="DigNum (严格)"("NumText.BGColor"=u32 16777215) -> ()  [unwired: 2 in, 2 out]
                n1405 = Select(t=0, s=w1830, f=1) -> (s? t:f=w1831:i32)
                n1406 = property on="一级故障 6" class="Clust (严格)"("DisabledEnum"=w1831) -> ()  [unwired: 2 in, 2 out]
                n1407 = global read "功能码全局.vi" "18"() -> (w1837:bool[])
                n1408 = Index Array(array=w1837, index #1=2 ("索引"), index #2=5 ("索引")) -> (element #1=w1835:bool, element #2=w1834:bool)
                n1409 = Not(x=w1828) -> (.not. x?=w1839:bool)
              }
              frame "SOC过低(2)", "电压不均衡(2)", "电压过低(2)", "电压过高(2)", "二级故障阀值", "温度不均衡(2)", "温度过低(2)", "温度过高(2)" {
                w1841 = FALSE ("1 6")
                n1410 = property on="从板号" class="DigNum (严格)"("NumText.BGColor"=u32 16777215) -> ()  [unwired: 2 in, 2 out]
                n1411 = Select(t=0, s=w1844, f=1) -> (s? t:f=w1843:i32)
                n1412 = property on="一级故障 7" class="Clust (严格)"("DisabledEnum"=w1843) -> ()  [unwired: 2 in, 2 out]
                n1413 = global read "功能码全局.vi" "18"() -> (w1850:bool[])
                n1414 = Index Array(array=w1850, index #1=3 ("索引"), index #2=6 ("索引")) -> (element #1=w1848:bool, element #2=w1847:bool)
                n1415 = Not(x=w1841) -> (.not. x?=w1852:bool)
              }
              frame "SOC过低(3)", "电压不均衡(3)", "电压过低(3)", "电压过高(3)", "三级故障阀值", "温度不均衡(3)", "温度过低(3)", "温度过高(3)" {
                w1854 = FALSE ("1 6")
                n1416 = property on="从板号" class="DigNum (严格)"("NumText.BGColor"=u32 16777215) -> ()  [unwired: 2 in, 2 out]
                n1417 = Select(t=0, s=w1857, f=1) -> (s? t:f=w1856:i32)
                n1418 = property on="一级故障 8" class="Clust (严格)"("DisabledEnum"=w1856) -> ()  [unwired: 2 in, 2 out]
                n1419 = global read "功能码全局.vi" "18"() -> (w1863:bool[])
                n1420 = Index Array(array=w1863, index #1=4 ("索引"), index #2=7 ("索引")) -> (element #1=w1861:bool, element #2=w1860:bool)
                n1421 = Not(x=w1854) -> (.not. x?=w1865:bool)
              }
              frame "快换参数" {
                w1867 = FALSE ("1 6")
                n1422 = Select(t=0, s=w1888, f=1) -> (s? t:f=w1887:i32)
                n1423 = property on="电池组信息" class="Clust (严格)"("Disabled"=w1887) -> ()  [unwired: 2 in, 2 out]
                n1424 = property on="从板号" class="DigNum (严格)"("NumText.BGColor"=u32 16777215) -> ()  [unwired: 2 in, 2 out]
                n1425 = global read "功能码全局.vi" "24"() -> (w1884:bool[])
                n1426 = global read "功能码全局.vi" "23"() -> (w1885:bool[])
